vi "Biometry Keratometric Parameter2String.vi"(8 "error in (no error)":errorcluster caption="错误输入（无错误）", 9 "Biometry Parameter":T2, 10 "Biometry State":T1, 11 "No":i32) -> (0 "error out":errorcluster caption="错误输出", 2 "Data Output":string[](array[string]))   [LabVIEW 2015, in "Utility VIs.lvlib"]
doc: "该模板用于创建子VI。"
uses:
  Utility VIs.lvlib
  Database Processing/Support/Table/Biometry Parameter.ctl
  Database Processing/Support/Table/Biometry State.ctl
  Database Processing/Database Processing.lvlib
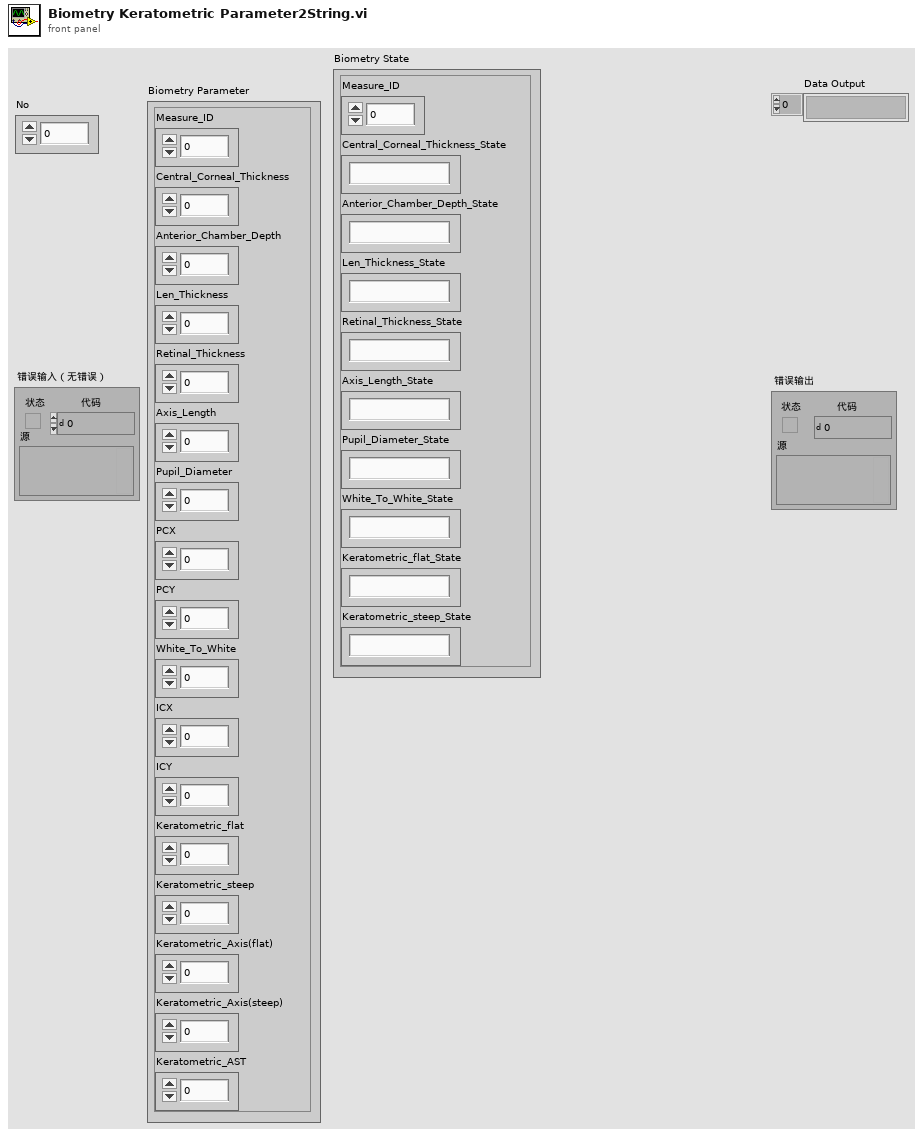
[diagram p1: front panel]
types:
  T1 = typedef "Database Processing.lvlib/Biometry State.ctl" = cluster{"Measure_ID":i64, "Central_Corneal_Thickness_State":string, "Anterior_Chamber_Depth_State":string, "Len_Thickness_State":string, "Retinal_Thickness_State":string, "Axis_Length_State":string, "Pupil_Diameter_State":string, "White_To_White_State":string, "Keratometric_flat_State":string, "Keratometric_steep_State":string}
  T2 = typedef "Database Processing.lvlib/Biometry Parameter.ctl" = cluster{"Measure_ID":i64, "Central_Corneal_Thickness":sgl, "Anterior_Chamber_Depth":sgl, "Len_Thickness":sgl, "Retinal_Thickness":sgl, "Axis_Length":sgl, "Pupil_Diameter":sgl, "PCX":sgl, "PCY":sgl, "White_To_White":sgl, "ICX":sgl, "ICY":sgl, "Keratometric_flat":sgl, "Keratometric_steep":sgl, "Keratometric_Axis(flat)":sgl, "Keratometric_Axis(steep)":sgl, "Keratometric_AST":sgl}
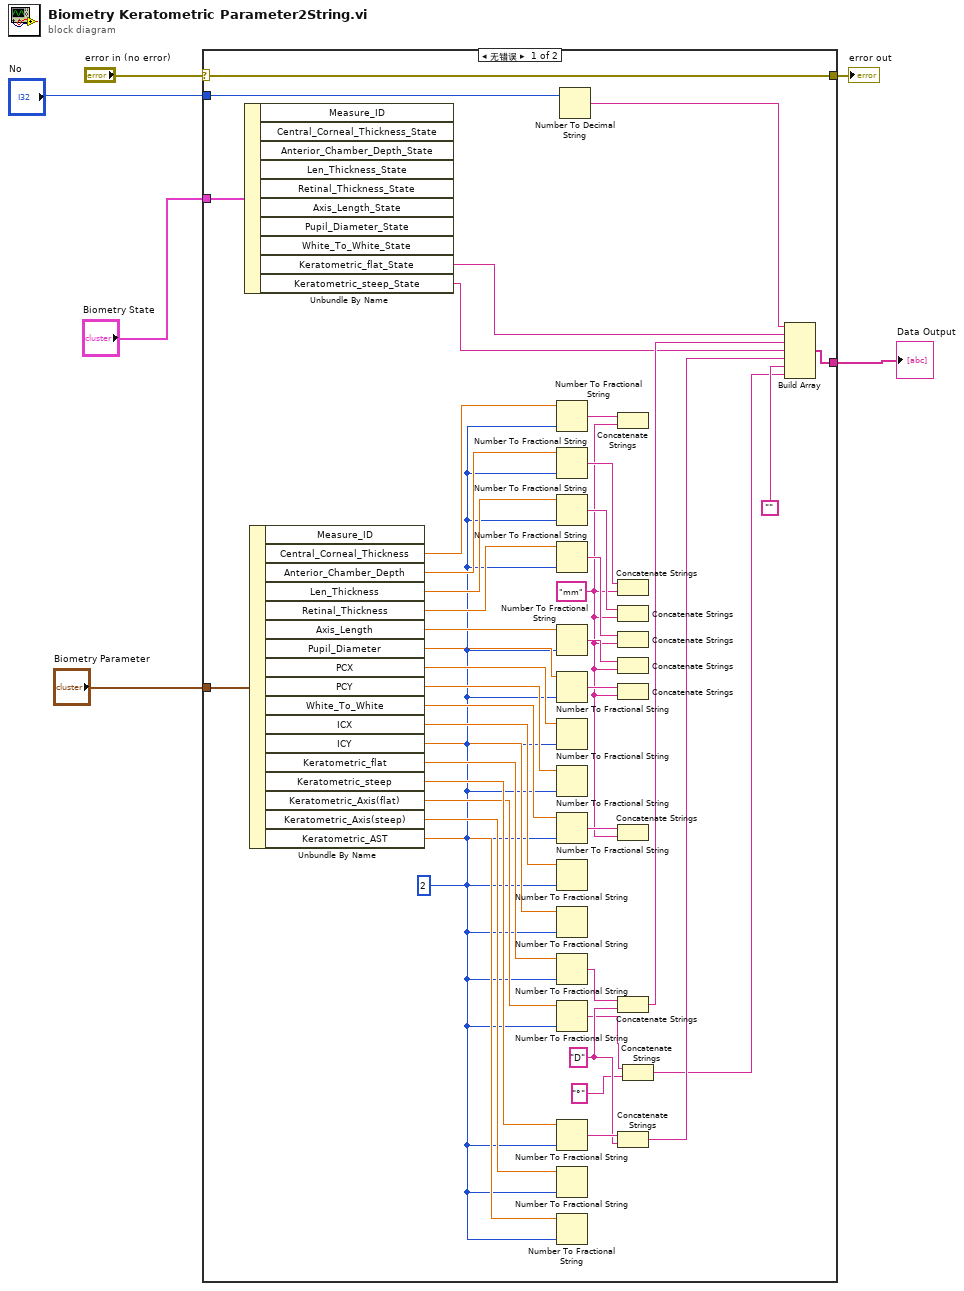
[diagram p0: block diagram]
diagram:
  n1 = case shown="无错误" "error in (no error)" {
    selector: "error in (no error)" -> [w18 w49]
    tunnel: [w18 w49] -> w5
    tunnel: "Biometry Parameter" -> [w48 _]
    tunnel: "Biometry State" -> [w47 _]
    tunnel: [w17 _] -> w2
    tunnel: "No" -> [w16 _]
    frame No Error {
      w22 = "D" ("字符串")
      w23 = "mm" ("字符串")
      w19 = i16 2 ("精度(6)")
      n2 = Unbundle By Name(w47) -> ("Keratometric_flat_State"=w14:string, "Keratometric_steep_State"=w7:string)  [unwired: 8 out]
      n3 = Unbundle By Name(w48) -> ("Central_Corneal_Thickness"=w46:sgl, "Anterior_Chamber_Depth"=w45:sgl, "Len_Thickness"=w44:sgl, "Retinal_Thickness"=w43:sgl, "Axis_Length"=w42:sgl, "Pupil_Diameter"=w41:sgl, "PCX"=w40:sgl, "PCY"=w39:sgl, "White_To_White"=w38:sgl, "ICX"=w37:sgl, "ICY"=w36:sgl, "Keratometric_flat"=w35:sgl, "Keratometric_steep"=w34:sgl, "Keratometric_Axis(flat)"=w33:sgl, "Keratometric_Axis(steep)"=w21:sgl, "Keratometric_AST"=w20:sgl)  [unwired: 1 out]
      n4 = Number To Fractional String(number=w46, precision (6)=w19) -> (F-format string=w32:string)  [unwired: 2 in]
      n5 = Number To Fractional String(number=w45, precision (6)=w19) -> (F-format string=w31:string)  [unwired: 2 in]
      n6 = Number To Fractional String(number=w44, precision (6)=w19) -> (F-format string=w30:string)  [unwired: 2 in]
      n7 = Number To Fractional String(number=w43, precision (6)=w19) -> (F-format string=w29:string)  [unwired: 2 in]
      n8 = Number To Fractional String(number=w42, precision (6)=w19) -> (F-format string=w28:string)  [unwired: 2 in]
      n9 = Number To Fractional String(number=w41, precision (6)=w19) -> (F-format string=w27:string)  [unwired: 2 in]
      n10 = Number To Fractional String(number=w40, precision (6)=w19) -> ()  [unwired: 2 in, 1 out]
      n11 = Number To Fractional String(number=w39, precision (6)=w19) -> ()  [unwired: 2 in, 1 out]
      n12 = Number To Fractional String(number=w38, precision (6)=w19) -> (F-format string=w26:string)  [unwired: 2 in]
      n13 = Number To Fractional String(number=w37, precision (6)=w19) -> ()  [unwired: 2 in, 1 out]
      n14 = Number To Fractional String(number=w36, precision (6)=w19) -> ()  [unwired: 2 in, 1 out]
      n15 = Number To Fractional String(number=w35, precision (6)=w19) -> (F-format string=w25:string)  [unwired: 2 in]
      n16 = Number To Fractional String(number=w33, precision (6)=w19) -> (F-format string=w9:string)  [unwired: 2 in]
      n17 = Number To Fractional String(number=w34, precision (6)=w19) -> (F-format string=w24:string)  [unwired: 2 in]
      n18 = Number To Fractional String(number=w21, precision (6)=w19) -> ()  [unwired: 2 in, 1 out]
      n19 = Number To Fractional String(number=w20, precision (6)=w19) -> ()  [unwired: 2 in, 1 out]
      n20 = Number To Decimal String(number=w16) -> (decimal integer string=w13:string)  [unwired: 1 in]
      n21 = Concatenate Strings(w32, w23) -> ()  [unwired: 1 out]
      n22 = Concatenate Strings(w31, w23) -> ()  [unwired: 1 out]
      n23 = Concatenate Strings(w30, w23) -> ()  [unwired: 1 out]
      n24 = Concatenate Strings(w29, w23) -> ()  [unwired: 1 out]
      n25 = Concatenate Strings(w28, w23) -> ()  [unwired: 1 out]
      n26 = Concatenate Strings(w27, w23) -> ()  [unwired: 1 out]
      n27 = Concatenate Strings(w26, w23) -> ()  [unwired: 1 out]
      n28 = Concatenate Strings(w25, w22) -> (w12:string)
      n29 = Concatenate Strings(w24, w22) -> (w11:string)
      n30 = Concatenate Strings(w9, "°" ("字符串")) -> (w8:string)
      n31 = Build Array(w13, w14, w12, w7, w11, "", w8) -> (w17:string[])
    }
    frame Error {
    }
  }
  "error out" <- w5
  "Data Output" <- w2
